vi "GEA2 Message Event Handler.vi"(4 "Data":refnum<user-event>, 5 "Event Data":T1, 6 "Control Ref":refnum<k24>, 7 "Event Common Data":T2) -> ()   [LabVIEW 2014, in "GEA2_Toolkit.lvlib"]
doc: "This subVI is executed upon receiving an event (GEA2 data). It parses the data and returns: source, destination, command, length, CRC, and data. The inputs CANNOT be modified."
uses:
  library/GEA2_Toolkit.lvlib
  C:/Automation/DLLs/PC Tools .NET/GeaCommunication.dll
  Automation/DLLs/PC Tools .NET/GeaCommunication.dll
  type defs/Data Out.ctl
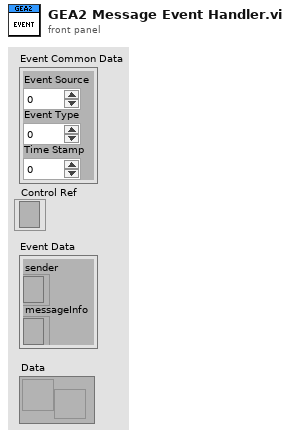
[diagram p1: front panel]
types:
  T1 = cluster{"sender":refnum<k24>, "messageInfo":refnum<k24>}
  T2 = cluster{"Event Source":i32, "Event Type":u32, "Time Stamp":u32}
  T3 = typedef "GEA2_Toolkit.lvlib/Data Out.ctl" = cluster{"Source":u8, "Destination":u8, "Command":u8, "Length":u8, "CRC":u16, "Message":string}
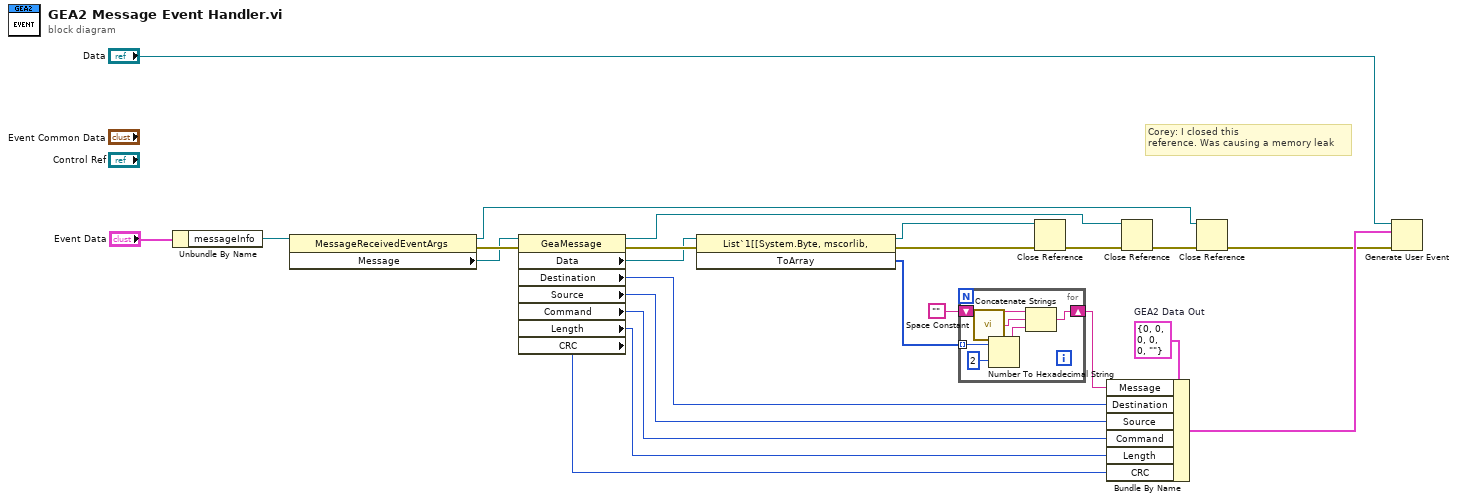
[diagram p0: block diagram]
diagram:
  w23 = T3 {"Source"=0, "Destination"=0, "Command"=0, "Length"=0, "CRC"=0, "Message"=""}  # GEA2 Data Out
  # "Corey: I closed this \nreference. Was causing a memory leak"
  n1 = Unbundle By Name("Event Data") -> ("messageInfo"=w18:refnum<k24>)
  n2 = property class="MessageReceivedEventArgs"(reference=w18) -> (reference out=w2:refnum<k24>, error out=w17:errorcluster, "Message"=w16:refnum<k24>)  [unwired: 1 in]
  n3 = property class="GeaMessage"(reference=w16, error in=w17) -> (reference out=w11:refnum<k24>, error out=w15:errorcluster, "Data"=w1:refnum<k24>, "Destination"=w22:u8, "Source"=w21:u8, "Command"=w20:u8, "Length"=w10:u8, "CRC"=w9:u16)
  n4 = invoke class="List`1[[System.Byte, mscorlib, " method="ToArray"(reference=w1, error in=w15) -> (reference out=w12:refnum<k24>, error out=w14:errorcluster, "ToArray"=w5:u8[])  [unwired: 1 in]
  n5 = for {
    tunnel: w5 -> [w30] mode=indexing
    shift-right: [w29] -> w7
    shift-left: "" -> [w28]
    n6 = call <vilib>:"Space Constant.vi"() -> ("String"=w25:string)
    n7 = Number To Hexadecimal String(1:i16 2 ("width (-)"), 2:w30) -> (0:w26:string)
    n8 = Concatenate Strings(w28, w25, w26) -> (w29:string)
  }
  n9 = Close Reference(reference=w12, error in (no error)=w14) -> (error out=w13:errorcluster)
  n10 = Bundle By Name(cluster=w23, "Message"=w7, "Destination"=w22, "Source"=w21, "Command"=w20, "Length"=w10, "CRC"=w9) -> (w19:T3)
  n11 = Close Reference(reference=w11, error in (no error)=w13) -> (error out=w4:errorcluster)
  n12 = Close Reference(reference=w2, error in (no error)=w4) -> (error out=w3:errorcluster)
  n13 = Generate User Event(user event="Data", event data cluster=w19, error in=w3) -> ()  [unwired: 1 in, 2 out]
